vi "Measurement.vi"(8 "error in (no error)":errorcluster, 9 "Grandeza":string, 10 "Multiplicador":dbl, 11 "U1252 in":refnum<class "U1252.lvclass">) -> (0 "error out":errorcluster, 2 "Measurement":dbl, 3 "U1252 out":refnum<class "U1252.lvclass">)   [LabVIEW 2015, in "U1252.lvclass"]
doc: "VI used to measure Value using the multimeter"
uses:
  U1252.lvclass
  <instrlib>/U1250 Series Multimeter Device Driver/U1250 Series Digital Multimeter.lvlib
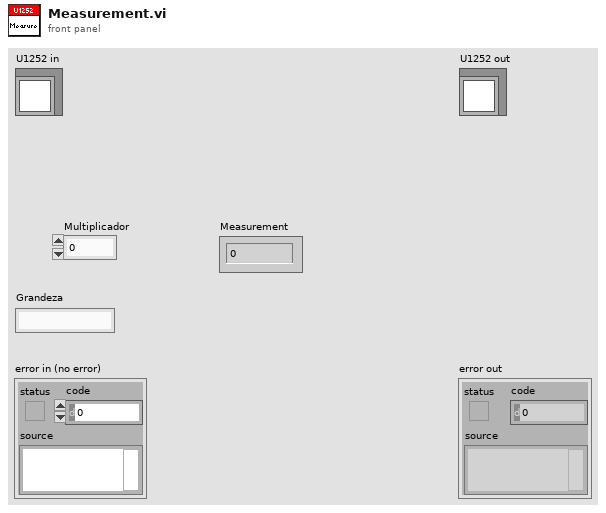
[diagram p1: front panel]
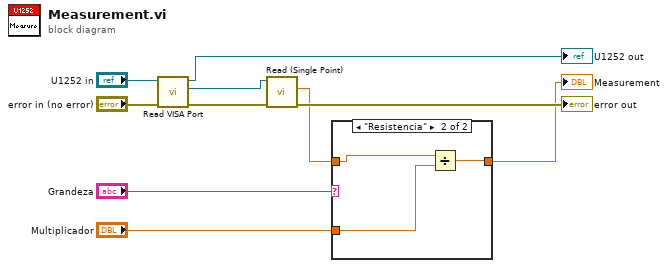
[diagram p0: block diagram]
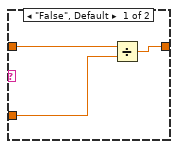
[diagram p2: hidden frame]
diagram:
  n1 = call-dynamic "Read VISA Port.vi"("error in (no error)"="error in (no error)", "Device in"="U1252 in") -> ("error out"=w6:errorcluster, "VISA Port"=w8:refnum<visa-resource-name>, "Device out"=→"U1252 out":refnum<class "U1252.lvclass">)  [unwired: 7 in]
  n2 = call <instrlib>:"Read (Single Point).vi"("error in (no error)"=w6, "VISA resource name"=w8) -> ("error out"=→"error out":errorcluster, "Measurement"=w2:dbl)  [unwired: 7 in, 1 out]
  n3 = case shown="\"Resistencia\"" "Grandeza" {
    tunnel: "Multiplicador" -> [w13 w14]
    tunnel: w2 -> [w12 w15]
    tunnel: [w11 w16] -> w1
    frame "False", Default {
      n4 = Divide(x=w12, y=w13) -> (x/y=w11:dbl)
    }
    frame "Resistencia" {
      n5 = Divide(x=w15, y=w14) -> (x/y=w16:dbl)
    }
  }
  "Measurement" <- w1
